vi "Start Module.vi"(6 "Show Main VI Diagram on Init (F)":bool, 7 "GenNet Protocol":refnum<class "GenNet Protocol.lvclass">, 8 "error in (no error)":errorcluster, 9 "Caller SystemMsg":refnum<user-event>, 10 "Caller MsgQ":refnum<class "DQMH-GenNet Message Queue.lvclass">, 11 "Run as Singleton? (F)":bool) -> (0 "error out":errorcluster, 1 "Wait for Event Sync?":bool, 2 "GenNet-Client Broadcast Events":T1, 3 "Module ID":i32)   [LabVIEW 2020, in "GenNet-Client.lvlib"]
doc: "Launches the Module Main.vi.\n____\nHAMPEL SOFTWARE ENGINEERING v3.8.0 (2023-12-18 14:41)"
uses:
  GenNet-Client.lvlib
  GenNet Protocols/GenNet Protocol.lvclass
  Broadcast Events--cluster.ctl
  Did Init Argument--cluster.ctl
  Status Updated Argument--cluster.ctl
  Error Reported Argument--cluster.ctl
  Stop Argument--cluster.ctl
  Get Module Execution Status Argument--cluster.ctl
  DQMH-GenNet Message Queue.lvclass
  hse-dqmh/Controls/System Message Argument--cluster.ctl
  hse-dqmh/Controls/System Message Source.ctl
  Module Running State--enum.ctl
  <vilib>/Delacor/Delacor QMH/Libraries/Cloneable Module Admin_class/Delacor_lib_QMH_Cloneable Module Admin.lvclass
  C:/Program Files (x86)/National Instruments/LabVIEW 2020/vi.lib/Delacor/Delacor QMH/Libraries/Module Admin_class/Delacor_lib_QMH_Module Admin.lvclass
  GenNet Protocols/Variant Protocol/GenNet Variant Protocol.lvclass
  C:/GitLab-Runner/builds/7NHnU7RQc/0/open-source/hse-libraries/Source/hse-gennet/GenNet Protocols/GenNet Protocol.lvclass
  VI Reference Management/Main VI Type--strict_vi_ref.ctl
  <vilib>/Delacor/Delacor QMH/Libraries/Cloneable Module Admin_class/Delacor_lib_QMH_Cloneable Module Admin.lvclass/Delacor_lib_QMH_Cloneable Module Admin.ctl
  <vilib>/Delacor/Delacor QMH/Libraries/Module Admin_class/Delacor_lib_QMH_Module Admin.lvclass/Delacor_lib_QMH_Module Admin.ctl
  <vilib>/Delacor/Delacor QMH/Libraries/Cloneable Module Admin_class/Delacor_lib_QMH_Set Module ID.vi
  <vilib>/Delacor/Delacor QMH/Libraries/Module Admin_class/Delacor_lib_QMH_Set External Launch.vi
  Main.vi
  <vilib>/Utility/error.llb/Error Cluster From Error Code.vi
  <vilib>/ErrorRing/Error Ring.xnode
  VI Reference Management/VI Reference Management.lvlib
  Clone Registration/Clone Registration.lvlib
  hse-dqmh/hse-dqmh.lvlib
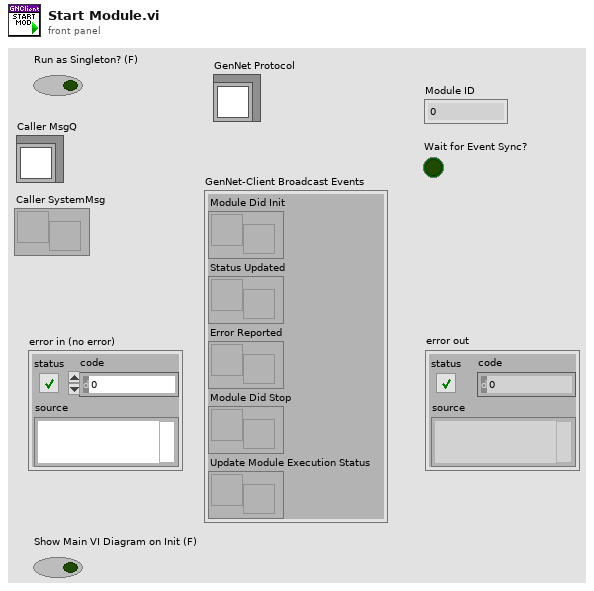
[diagram p1: front panel]
types:
  T1 = typedef "GenNet-Client.lvlib/Broadcast Events--cluster.ctl" = cluster{"Module Did Init":refnum<user-event>, "Status Updated":refnum<user-event>, "Error Reported":refnum<user-event>, "Module Did Stop":refnum<user-event>, "Update Module Execution Status":refnum<user-event>}
  T2 = typedef "GenNet-Client.lvlib/Module Running State--enum.ctl" = enum16{"Not Running", "Running as Cloneable", "Running as Singleton"}
  T3 = enum32{"Bad", "Idle", "Run top level", "Running"}
  T4 = typedef "GenNet-Client.lvlib/VI Reference Management.lvlib/Main VI Type--strict_vi_ref.ctl" = refnum<vi>
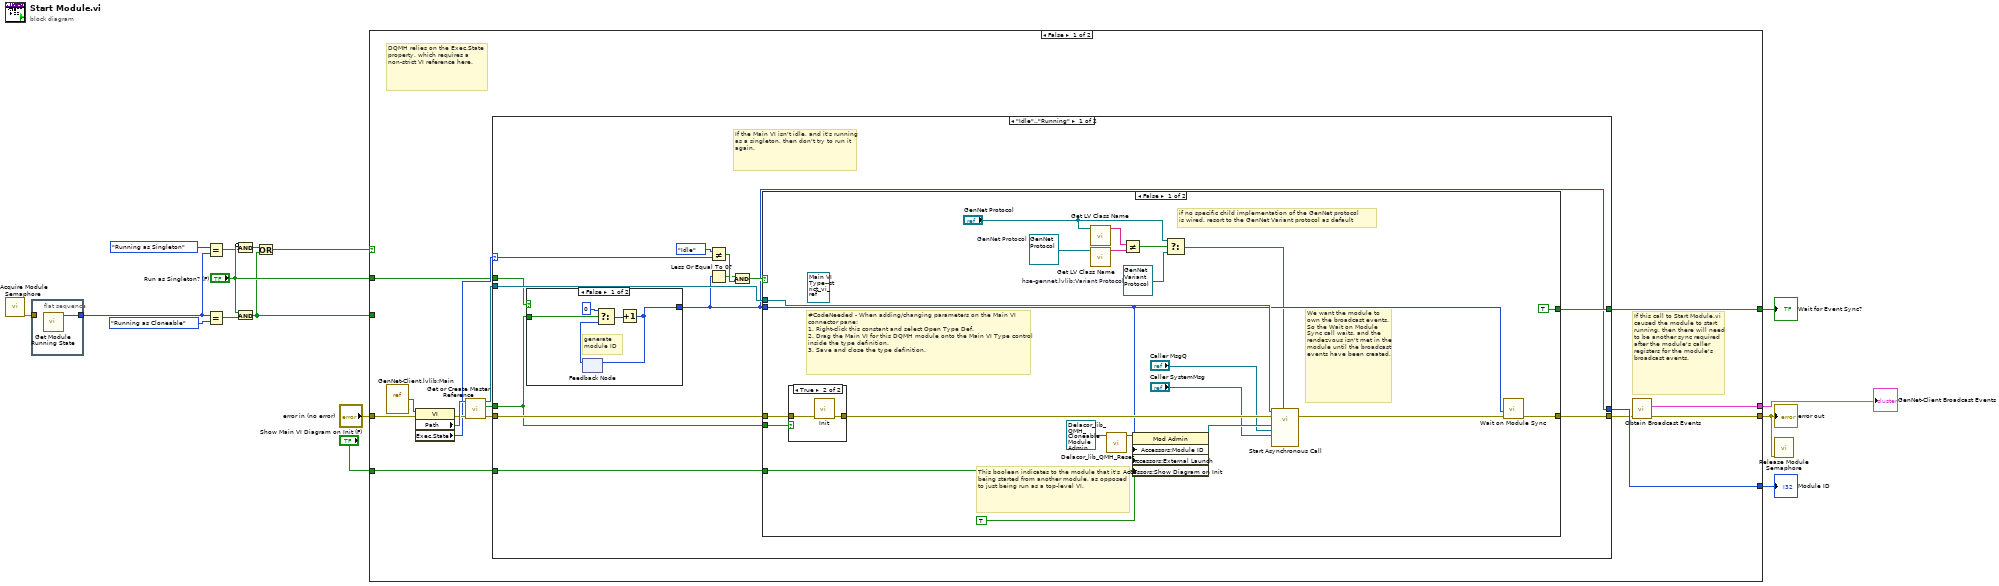
[diagram p0: block diagram]
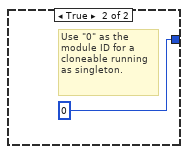
[diagram p2: hidden frame]
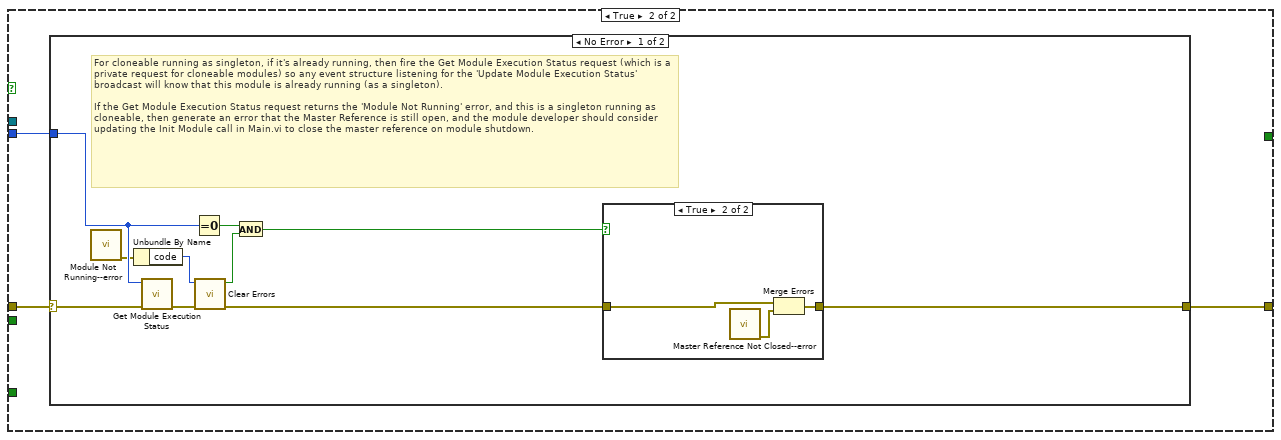
[diagram p4: hidden frame]
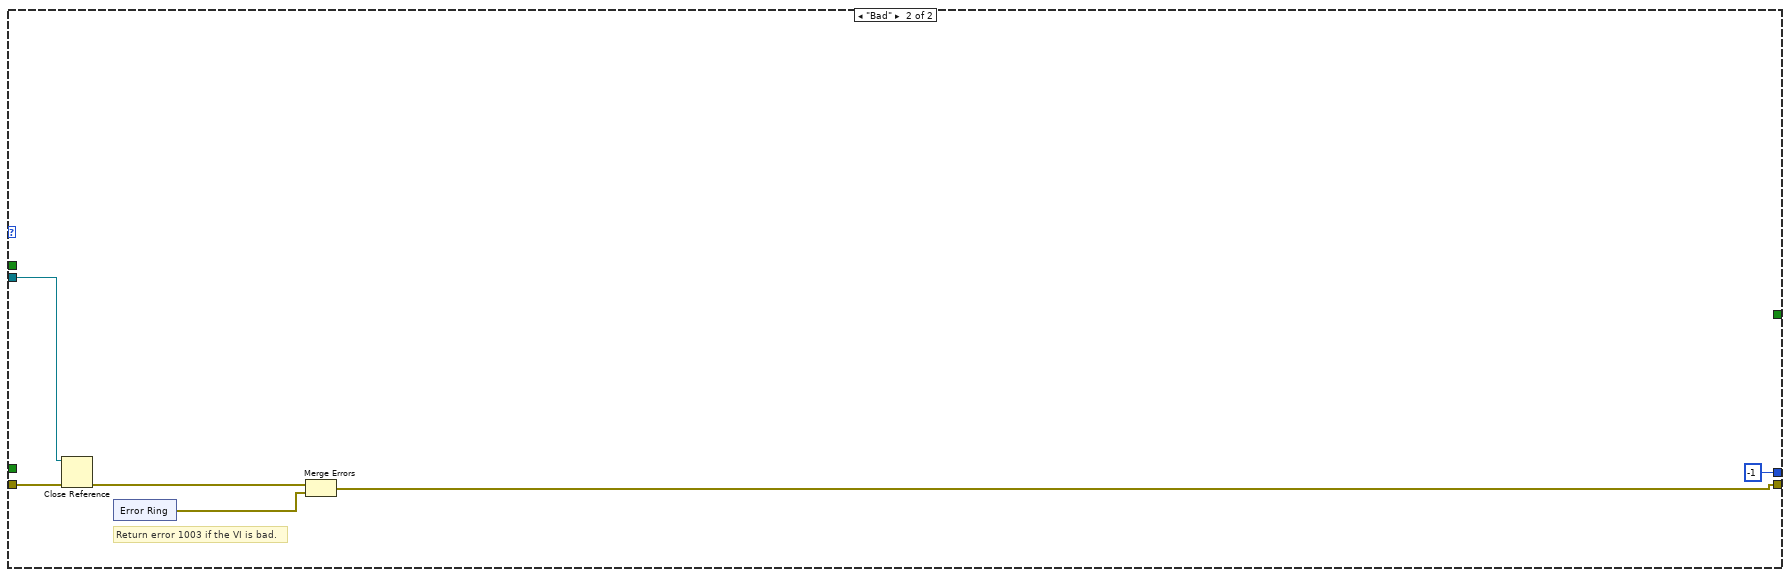
[diagram p7: hidden frame]
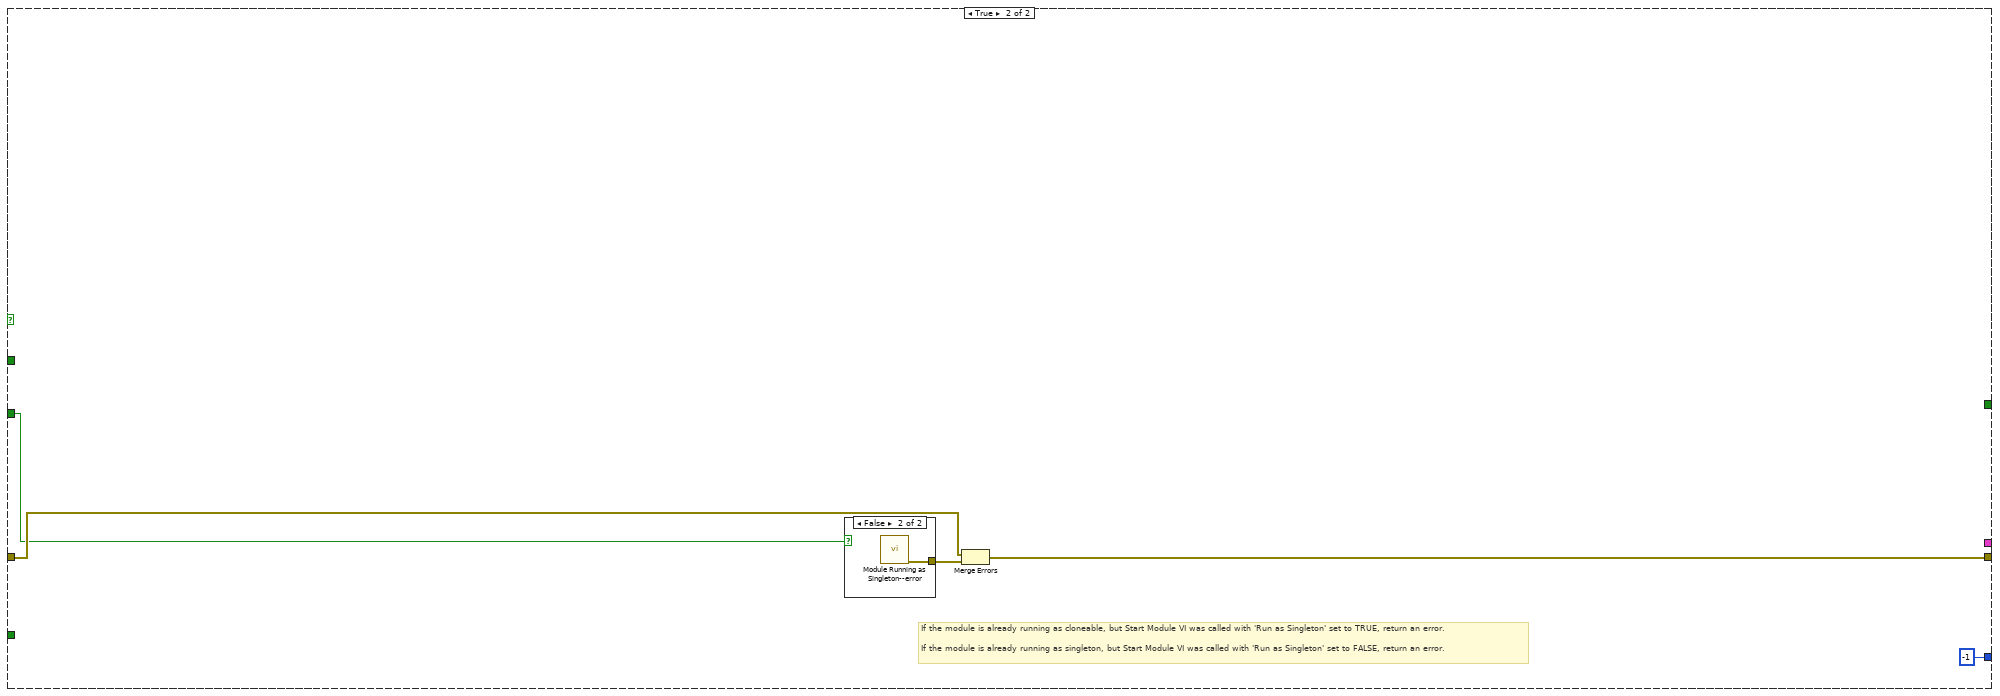
[diagram p8: hidden frame]
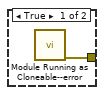
[diagram p9: hidden frame]
diagram:
  n1 = call "Acquire Module Semaphore.vi"() -> ("error out"=w3:errorcluster)  [unwired: 11 in]
  n2 = flat-sequence {
    tunnel: [w17] -> w4
    tunnel: w3 -> [_]
    frame #0 {
      n3 = call "Get Module Running State.vi"() -> ("Module Running State"=w17:T2)  [unwired: 11 in]
    }
  }
  n4 = Equal?(x=Module_Running_State--enum."Running as Singleton" ("DQMH_SINGLETON_ENUM"), y=w4) -> (x = y?=w7:bool)
  n5 = Equal?(x=w4, y=Module_Running_State--enum."Running as Cloneable" ("DQMH_CLONEABLE_ENUM")) -> (x = y?=w11:bool)
  n6 = And(x="Run as Singleton? (F)", y=w11) -> (x .and. y?=w5:bool)
  n7 = Compound Arithmetic op=AND(invert "Run as Singleton? (F)", w7) -> (w9:bool)
  n8 = Or(x=w9, y=w5) -> (x .or. y?=w10:bool)
  n9 = case shown="False" w10 {
    tunnel: "error in (no error)" -> [w32 w109]
    tunnel: [w21 w108] -> w2
    tunnel: [w20 _] -> w15
    tunnel: [w31 _] -> w14
    tunnel: [w27 -1] -> w13
    tunnel: "Run as Singleton? (F)" -> [w24 _]
    tunnel: w5 -> [_ w105]
    tunnel: "Show Main VI Diagram on Init (F)" -> [w18 _]
    frame False {
      # "DQMH relies on the Exec.State property, which requires a non-strict VI reference here."
      # "If this call to Start Module.vi caused the module to start running, then there will need to be another sync required after the module's caller registers for the module's broadcast events."
      n10 = vi-ref "GenNet-Client.lvlib:Main.vi"() -> (w19:refnum<vi>)
      n11 = property class="VI"(reference=w19, error in=w32) -> (error out=w29:errorcluster, "Path"=w30:path, "Exec.State"=w25:T3)  [unwired: 1 out]
      n12 = call "Get or Create Master Reference.vi"("error in (no error)"=w29, "Main VI Path"=w30) -> ("error out"=w28:errorcluster, "New Reference Created"=w23:bool, "Master Reference"=w26:T4)  [unwired: 7 in]
      n13 = case shown="\"Idle\"..\"Running\"" w25 {
        selector: w25 -> [w41 _]
        tunnel: w28 -> [w45 w100]
        tunnel: w26 -> [w43 w99]
        tunnel: [w42 w97] -> w22
        tunnel: [w44 _] -> w31
        tunnel: [w36 -1] -> w27
        tunnel: w24 -> [w35 _]
        tunnel: w23 -> [w34 _]
        tunnel: w18 -> [w33 _]
        frame "Idle".."Running" {
          # "If the Main VI isn't idle, and it's running as a singleton, then don't try to run it again."
          n14 = case shown="False" w35 {
            tunnel: [w50 0] -> w36
            tunnel: w34 -> [w46 _]
            frame False {
              # "generate module ID"
              n15 = feedback #1() -> (w48:i32)  [unwired: 1 in]
              n16 = Select(t=0, s=w46, f=w48) -> (s? t:f=w49:i32)
              n17 = Increment(x=w49) -> (x+1=w50:i32)
              n18 = feedback-in #1(w50) -> ()
            }
            frame True {
              # "Use \"0\" as the module ID for a cloneable running as singleton."
            }
          }
          n19 = Not Equal?(x=T3."Idle", y=w41) -> (x != y?=w39:bool)
          n20 = Less Or Equal To 0?(x=w36) -> (x <= 0?=w37:bool)
          n21 = And ("DQMH_AND")(x=w37, y=w39) -> (x .and. y?=w38:bool)
          n22 = case shown="False" w38 {
            tunnel: w45 -> [w68 w79]
            tunnel: [TRUE _] -> w44
            tunnel: w43 -> [w67 _]
            tunnel: [w64 w78] -> w42
            tunnel: w36 -> [w63 w77]
            tunnel: w34 -> [w62 _]
            tunnel: w33 -> [w52 _]
            frame False {
              w59 = refnum<class "GenNet Protocol.lvclass"> refnum  # GenNet Protocol
              w54 = refnum<class "GenNet Variant Protocol.lvclass"> refnum  # hse-gennet.lvlib:Variant Protocol
              (unwired) T4 refnum ("DQMH_STRICT_VIREF_TYPEDEF")
              # "if no specific child implementation of the GenNet protocol \nis wired, resort to the GenNet Variant protocol as default"
              # "#CodeNeeded - When adding/changing parameters on the Main VI connector pane:\n1. Right-click this constant and select Open Type Def.\n2. Drag the Main VI for this DQMH module onto the Main VI Type control inside the type definition.\n3. Save and close the type definition."
              # "We want the module to own the broadcast events. So the Wait on Module Sync call waits, and the rendezvous isn't met in the module until the broadcast events have been created."
              # "This boolean indicates to the module that it's being started from another module, as opposed to just being run as a top-level VI."
              n23 = case shown="True" w62 {
                tunnel: [w74 w76] -> w69
                tunnel: w68 -> [w74 w75]
                frame False {
                }
                frame True {
                  n24 = call "Init.vi"("error in (no error)"=w75) -> ("error out"=w76:errorcluster)  [unwired: 7 in, 3 out]
                }
              }
              n25 = call <vilib>:"Get LV Class Name.vi"("object"="GenNet Protocol") -> ("class name"=w58:string)  [unwired: 9 in, 1 out]
              n26 = call <vilib>:"Get LV Class Name.vi"("object"=w59) -> ("class name"=w57:string)  [unwired: 9 in, 1 out]
              n27 = call-dynamic "Delacor_lib_QMH_Reset.vi"("Mod Admin in"=refnum<class "Delacor_lib_QMH_Cloneable Module Admin.lvclass"> refnum) -> ("Mod Admin out"=w72:refnum<class "Delacor_lib_QMH_Cloneable Module Admin.lvclass">)  [unwired: 9 in, 1 out]
              n28 = Not Equal?(x=w58, y=w57) -> (x != y?=w56:bool)
              n29 = property class="Mod Admin"(reference=w72, "Accessors:Module ID"=w63, "Accessors:External Launch"=TRUE ("DQMH_EXTERNAL_LAUNCH"), "Accessors:Show Diagram on Init"=w52) -> (reference out=w66:refnum<class "Delacor_lib_QMH_Cloneable Module Admin.lvclass">)  [unwired: 1 in, 1 out]
              n30 = Select(t="GenNet Protocol", s=w56, f=w54) -> (s? t:f=w53:refnum<class "GenNet Protocol.lvclass">)
              n31 = call-by-ref "Start Asynchronous Call"(reference=w67, error in=w69, "GenNet Protocol"=w53, "Caller SystemMsg"="Caller SystemMsg", "Caller MsgQ"="Caller MsgQ", "Module Admin"=w66) -> (error out=w65:errorcluster)  [unwired: 8 in, 1 out]
              n32 = call "Wait on Module Sync.vi"("error in (no error)"=w65, "Module ID"=w63) -> ("error out"=w64:errorcluster)  [unwired: 9 in]
            }
            frame True {
              n33 = case shown="No Error" w79 {
                selector: w79 -> [w89 w94]
                tunnel: [w80 w94] -> w78
                tunnel: w77 -> [w87 _]
                frame No Error {
                  # "For cloneable running as singleton, if it's already running, then fire the Get Module Execution Status request (which is a private request for cloneable modules) so any event structure listening for the 'Update Module Execution Status' broadcast will know that this module is already running (as a singleton).\n\nIf the Get Module Execution Status request returns the 'Module Not Running' error, and this is a singleton running as cloneable, then generate an error that the Master Reference is still open, and the module developer should consider updating the Init Module call in Main.vi to close the master reference on module shutdown."
                  n34 = call "Module Not Running--error.vi"() -> ("error out"=w86:errorcluster)  [unwired: 11 in]
                  n35 = Unbundle By Name(w86) -> ("code"=w85:i32)
                  n36 = call "Get Module Execution Status.vi"("error in (no error)"=w89, "Module ID"=w87) -> ("error out"=w88:errorcluster)  [unwired: 9 in]
                  n37 = Equal To 0?(x=w87) -> (x = 0?=w83:bool)
                  n38 = call <vilib>:"Clear Errors.vi"("error in (no error)"=w88, "specific error code to clear (0: all)"=w85) -> ("error out"=w82:errorcluster, "specific error cleared?"=w84:bool)  [unwired: 4 in]
                  n39 = And(x=w83, y=w84) -> (x .and. y?=w81:bool)
                  n40 = case shown="True" w81 {
                    tunnel: w82 -> [w90 w93]
                    tunnel: [w90 w92] -> w80
                    frame False {
                    }
                    frame True {
                      n41 = call "Master Reference Not Closed--error.vi"() -> ("error out"=w91:errorcluster)  [unwired: 11 in]
                      n42 = Merge Errors(w93, w91) -> (w92:errorcluster)
                    }
                  }
                }
                frame Error {
                }
              }
            }
          }
        }
        frame "Bad" {
          # "Return error 1003 if the VI is bad."
          n43 = Close Reference(reference=w99, error in (no error)=w100) -> (error out=w98:errorcluster)
          n44 = xnode "Error Ring"() -> ("error out"=w96:errorcluster)
          n45 = Merge Errors(w98, w96) -> (w97:errorcluster)
        }
      }
      n46 = call "Obtain Broadcast Events.vi"("error in (no error)"=w22) -> ("error out"=w21:errorcluster, "GenNet-Client Broadcast Events"=w20:T1)  [unwired: 9 in]
    }
    frame True {
      # "If the module is already running as cloneable, but Start Module VI was called with 'Run as Singleton' set to TRUE, return an error.\n\nIf the module is already running as singleton, but Start Module VI was called with 'Run as Singleton' set to FALSE, return an error."
      n47 = case shown="False" w105 {
        tunnel: [w110 w111] -> w106
        frame True {
          n48 = call "Module Running as Cloneable--error.vi"() -> ("error out"=w110:errorcluster)  [unwired: 11 in]
        }
        frame False {
          n49 = call "Module Running as Singleton--error.vi"() -> ("error out"=w111:errorcluster)  [unwired: 11 in]
        }
      }
      n50 = Merge Errors(w109, w106) -> (w108:errorcluster)
    }
  }
  "error out" <- w2
  "GenNet-Client Broadcast Events" <- w15
  "Wait for Event Sync?" <- w14
  "Module ID" <- w13
  n51 = call "Release Module Semaphore.vi"("error in (no error)"=w2) -> ()  [unwired: 10 in, 1 out]
